vi "Test FTDI SPI BASE AB-Set.vi"() -> ()   [LabVIEW 2018]
uses:
  PROJEKT/NIKO/Labview/Niko V4/FTDI SPI/Ctl/Sub Addr.ctl
panel:
  in  "nCS":u8 max=2 step=1
  in  "Set Channel":u16(ring) items=["Ch-A", "Ch-B"]
  in  "Ch-B (1-8)":bool[](array[boolean])=[FALSE, FALSE, FALSE, FALSE, FALSE, FALSE, FALSE, FALSE, FALSE, FALSE]
  out "Latch Reg":u16 format="%b"
  in  "Addr":T1 items=["Addr-0", "Addr-1", "Addr-2", "Addr-3", "Addr-4", "Addr-5", "Addr-6", "Addr-7"]
  out "error out":errorcluster
  in  "Ch-A(1-8)":bool[](array[boolean])=[FALSE, FALSE, FALSE, FALSE, FALSE, FALSE, FALSE, FALSE, FALSE, FALSE]
  out "Ini Status":bool
  in  "config":T2={"ClockRate"=50000, "LatencyTimer"=10, "configOptions 24-31"=0, "configOptions 16-23"=0, "configOptions 8-15"=0, "configOptions 0-7"=32, "Pin"=0, "reserved"=0} {"configOptions 24-31" format="%x"; "configOptions 16-23" format="%x"; "configOptions 8-15" format="%x"; "configOptions 0-7" format="%x"}
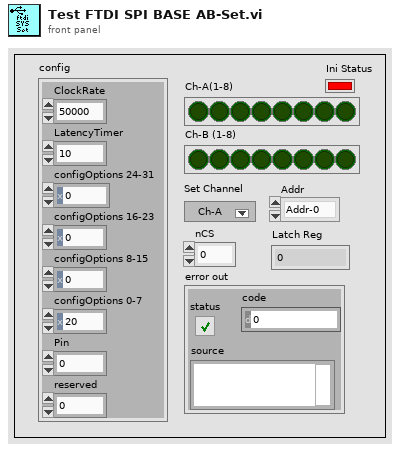
[diagram p1: front panel]
types:
  T1 = typedef "Sub Addr.ctl" = u16
  T2 = cluster{"ClockRate":u32, "LatencyTimer":u8, "configOptions 24-31":i8, "configOptions 16-23":i8, "configOptions 8-15":i8, "configOptions 0-7":u32, "Pin":u32, "reserved":u16}
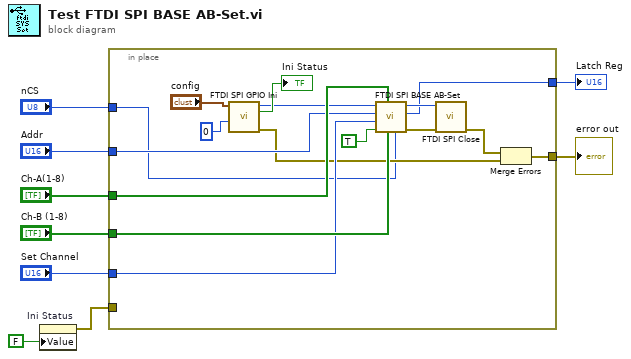
[diagram p0: block diagram]
diagram:
  n1 = property on="Ini Status" class="Bool (strict)"("Value"=FALSE ("Ini Status")) -> (error out=w6:errorcluster)  [unwired: 2 in, 1 out]
  n2 = in-place {
    in-place-border: "Addr" -> [w15]
    in-place-border: "Ch-A(1-8)" -> [w21]
    in-place-border: w6 -> [_]
    in-place-border: [w17] -> w5
    in-place-border: "Ch-B (1-8)" -> [w20]
    in-place-border: [w16] -> w3
    in-place-border: "Set Channel" -> [w14]
    in-place-border: "nCS" -> [w10]
    n3 = call "FTDI SPI GPIO Ini.vi"("Channel Nmb"=u8 0 ("FTDI Dev Nmb"), "config"="config") -> ("error out"=w13:errorcluster, "Ini Status"=→"Ini Status":bool, "handle out"=w12:u32)  [unwired: 5 in, 2 out]
    n4 = call "FTDI SPI BASE AB-Set.vi"("nCS"=w10, "Set Out-B (0-7)"=w20, "Set Out-A (0-7)"=w21, "Use Extra"=TRUE, "Set Channel"=w14, "Addr"=w15, "Handler In"=w12) -> ("error out"=w19:errorcluster, "Latch Reg"=w17:u32, "Handler Out"=w18:u32)  [unwired: 2 in]
    n5 = call "FTDI SPI Close.vi"("error in (no error)"=w19, "Handler In"=w18) -> ("error out"=w23:errorcluster)  [unwired: 9 in]
    n6 = Merge Errors(w23, w13) -> (w16:errorcluster)
  }
  "Latch Reg" <- w5
  "error out" <- w3
